vi "Enqueue Enum.vi"   [LabVIEW 2020, in "Enum Queue State Machine.lvlib"]
uses:
  Enum Queue State Machine.lvlib
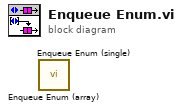
[diagram p0: block diagram]
diagram:
  n1 = call "Enqueue Enum (array).vi"() -> ()  [unwired: 10 in, 2 out]
  n2 = call "Enqueue Enum (single).vi"() -> ()  [unwired: 10 in, 2 out]
